vi "Translation Ctrl.vi"(0 "Alpha":dbl, 1 "Filtered Speed Y":dbl, 2 "Y In":dbl, 5 "Filtered Speed X":dbl, 7 "X In":dbl, 9 "X Desired":dbl, 11 "Original Difference X":dbl, 12 "Original Difference Y":dbl, 13 "Y Desired":dbl) -> (4 "Left":bool, 6 "Right":bool, 8 "Down":bool, 10 "Up":bool, 15 "Maneuver Complete?":bool)   [LabVIEW 2012]
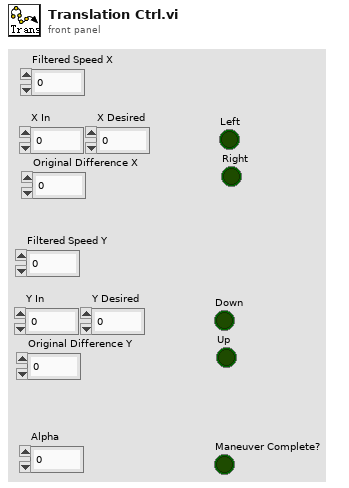
[diagram p1: front panel]
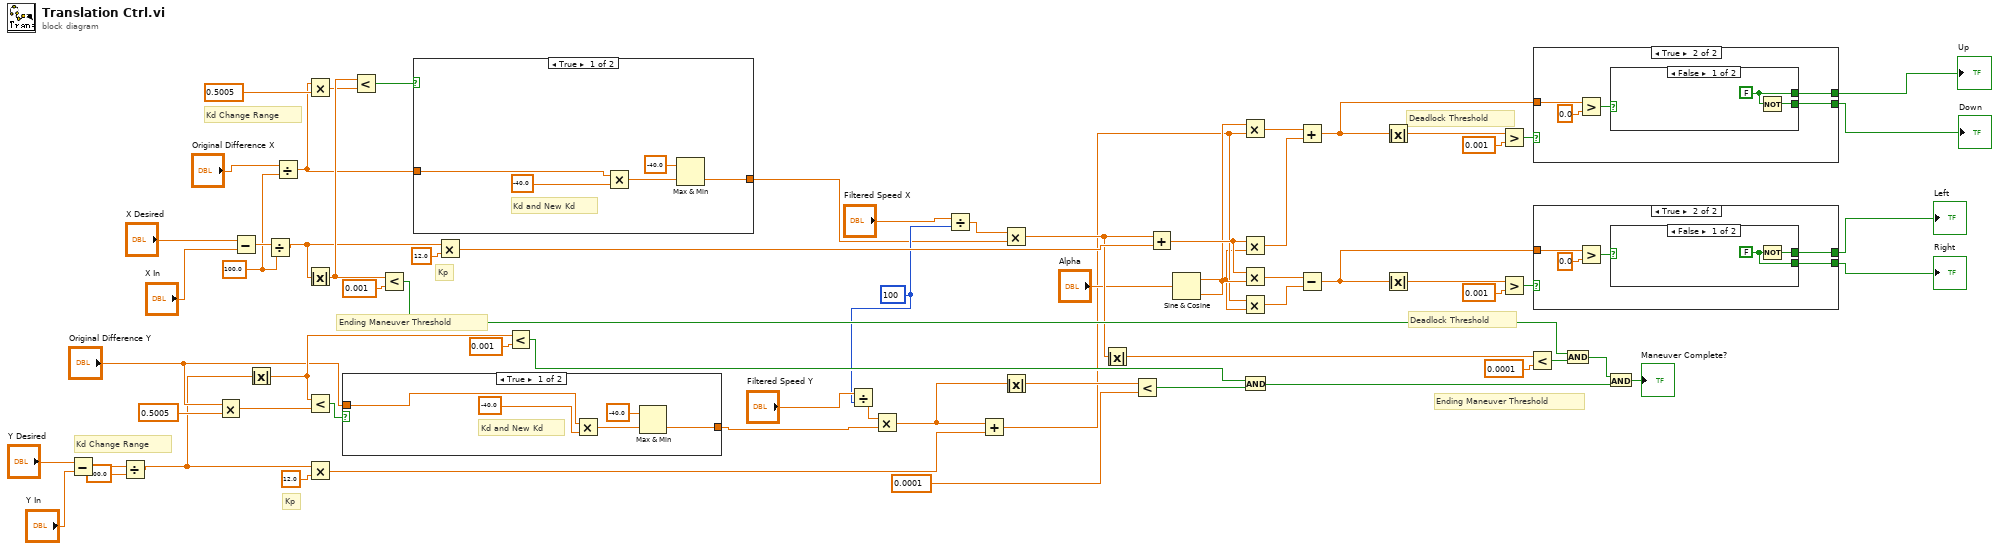
[diagram p0: block diagram]
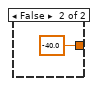
[diagram p2: hidden frame]
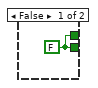
[diagram p3: hidden frame]
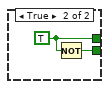
[diagram p4: hidden frame]
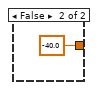
[diagram p5: hidden frame]
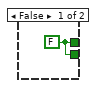
[diagram p6: hidden frame]
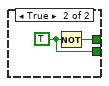
[diagram p7: hidden frame]
diagram:
  w8 = 100
  w12 = 100.0 ("y")
  # "Deadlock Threshold"
  # "Ending Maneuver Threshold"
  # "Kp"
  # "Kd Change Range"
  # "Deadlock Threshold"
  # "Ending Maneuver Threshold"
  # "Kp"
  # "Kd Change Range"
  n1 = Subtract(x="Y Desired", y="Y In") -> (x-y=w17:dbl)
  n2 = Divide(x=w17, y=100.0) -> (x/y=w15:dbl)
  n3 = Multiply(x="Original Difference Y", y=0.5005) -> (x*y=w37:dbl)
  n4 = Subtract(x="X Desired", y="X In") -> (x-y=w19:dbl)
  n5 = Absolute Value(x=w15) -> (abs(x)=w39:dbl)
  n6 = Divide(x=w19, y=w12) -> (x/y=w18:dbl)
  n7 = Divide(x="Original Difference X", y=w12) -> (x/y=w14:dbl)
  n8 = Multiply(x=w14, y=0.5005) -> (x*y=w55:dbl)
  n9 = Absolute Value(x=w18) -> (abs(x)=w57:dbl)
  n10 = Less?(x=w39, y=w37) -> (x < y?=w36:bool)
  n11 = Multiply(x=w15, y=12.0) -> (x*y=w49:dbl)
  n12 = case shown="True" w36 {
    tunnel: [w69 -40.0 ("y")] -> w5
    tunnel: "Original Difference Y" -> [w72 _]
    frame True {
      # "Kd and New Kd"
      n13 = Multiply(x=w72, y=-40.0) -> (x*y=w71:dbl)
      n14 = Max & Min(x=-40.0 ("y"), y=w71) -> (min(x,y)=w69:dbl)  [unwired: 1 out]
    }
    frame False {
    }
  }
  n15 = Less?(x=w57, y=w55) -> (x < y?=w54:bool)
  n16 = Less?(x=w57, y=0.001) -> (x < y?=w63:bool)
  n17 = case shown="True" w54 {
    tunnel: [w75 -40.0 ("y")] -> w6
    tunnel: w14 -> [w78 _]
    frame True {
      # "Kd and New Kd"
      n18 = Multiply(x=w78, y=-40.0) -> (x*y=w77:dbl)
      n19 = Max & Min(x=-40.0 ("y"), y=w77) -> (min(x,y)=w75:dbl)  [unwired: 1 out]
    }
    frame False {
    }
  }
  n20 = Multiply(x=w18, y=12.0) -> (x*y=w67:dbl)
  n21 = Less?(x=w39, y=0.001) -> (x < y?=w45:bool)
  n22 = Divide(x="Filtered Speed Y", y=w8) -> (x/y=w7:dbl)
  n23 = Multiply(x=w7, y=w5) -> (x*y=w44:dbl)
  n24 = Divide(x="Filtered Speed X", y=w8) -> (x/y=w10:dbl)
  n25 = Add(x=w44, y=w49) -> (x+y=w24:dbl)
  n26 = Multiply(x=w10, y=w6) -> (x*y=w62:dbl)
  n27 = Absolute Value(x=w44) -> (abs(x)=w43:dbl)
  n28 = Absolute Value(x=w62) -> (abs(x)=w61:dbl)
  n29 = Less?(x=w43, y=0.0001) -> (x < y?=w41:bool)
  n30 = Add(x=w62, y=w67) -> (x+y=w26:dbl)
  n31 = Sine & Cosine(0:"Alpha") -> (1:w23:dbl, 2:w25:dbl)
  n32 = Multiply(x=w25, y=w24) -> (x*y=w28:dbl)
  n33 = Multiply(x=w26, y=w23) -> (x*y=w29:dbl)
  n34 = Multiply(x=w26, y=w25) -> (x*y=w22:dbl)
  n35 = Multiply(x=w24, y=w23) -> (x*y=w21:dbl)
  n36 = And(x=w45, y=w41) -> (x .and. y?=w32:bool)
  n37 = Add(x=w28, y=w29) -> (x+y=w30:dbl)
  n38 = Subtract(x=w22, y=w21) -> (x-y=w27:dbl)
  n39 = Absolute Value(x=w30) -> (abs(x)=w48:dbl)
  n40 = Absolute Value(x=w27) -> (abs(x)=w66:dbl)
  n41 = Greater?(x=w48, y=0.001 ("x")) -> (0:w47:bool)
  n42 = Greater?(x=w66, y=0.001 ("x")) -> (0:w65:bool)
  n43 = Less?(x=w61, y=0.0001) -> (x < y?=w59:bool)
  n44 = case shown="True" w47 {
    tunnel: [w81 w86] -> w3
    tunnel: [w81 w84] -> w4
    tunnel: w30 -> [_ w83]
    frame False {
      w81 = FALSE
    }
    frame True {
      n45 = Greater?(x=w83, y=0.0) -> (0:w85:bool)
      n46 = case shown="False" w85 {
        tunnel: [w88 w90] -> w86
        tunnel: [w87 w89] -> w84
        frame False {
          w88 = FALSE ("clkwis")
          n47 = Not(x=w88) -> (.not. x?=w87:bool)
        }
        frame True {
          w90 = TRUE ("clkwis")
          n48 = Not(x=w90) -> (.not. x?=w89:bool)
        }
      }
    }
  }
  "Down" <- w4
  "Up" <- w3
  n49 = case shown="True" w65 {
    tunnel: [w91 w96] -> w2
    tunnel: [w91 w94] -> w1
    tunnel: w27 -> [_ w93]
    frame False {
      w91 = FALSE
    }
    frame True {
      n50 = Greater?(x=w93, y=0.0) -> (0:w95:bool)
      n51 = case shown="False" w95 {
        tunnel: [w98 w100] -> w96
        tunnel: [w97 w99] -> w94
        frame False {
          w98 = FALSE ("clkwis")
          n52 = Not(x=w98) -> (.not. x?=w97:bool)
        }
        frame True {
          w100 = TRUE ("clkwis")
          n53 = Not(x=w100) -> (.not. x?=w99:bool)
        }
      }
    }
  }
  "Left" <- w1
  "Right" <- w2
  n54 = And(x=w63, y=w59) -> (x .and. y?=w33:bool)
  n55 = And(x=w33, y=w32) -> (x .and. y?=→"Maneuver Complete?":bool)
